vi "MatrixSwitch.vi"(8 "error in (no error)":errorcluster, 10 "Action":T1(ring), 11 "Pickering in":refnum<class "PickeringPrague.lvclass">) -> (0 "error out":errorcluster, 2 "Continue?":bool, 3 "Pickering out":refnum<class "PickeringPrague.lvclass">)   [LabVIEW 2018, in "PickeringPrague.lvclass"]
uses:
  PickeringPrague.lvclass
  InstrumentSetup.vi
  InstrControl.lvclass
panel:
  out "Display Matrix":bool[][](array[boolean])
  # "Pickering Matrix Settings"
  # "X1"
  # "X2"
  # "X3"
  # "X4"
  # "X5"
  # "X6"
  # "X7"
  # "X8"
  # "X9"
  # "X10"
  # "X11"
  # "X12"
  # "Y1"
  # "Y2"
  # "Y3"
  # "Y4"
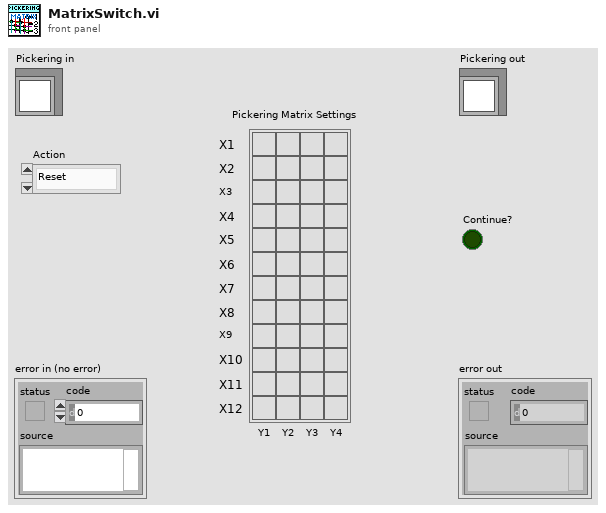
[diagram p1: front panel]
types:
  T1 = enum16{"Reset", "Ground", "Striptest SMU", "Striptest LCR", "IV", "CV", "Interstrip Cap", "Interstrip Res"}
  T2 = cluster{"Matrix address":string, "Mux1 address":string, "Mux2 address":string, "Matrix used?":bool, "Matrix X Channels":cluster{"LCR LO":i32, "LCR HI":i32, "SMU LO":i32, "SMU HI":i32, "GND":i32}, "Matrix Y Channels":cluster{"Flying Probe":i32, "Needle":i32}, "PickeringPrague.lvclass":refnum<class "PickeringPrague.lvclass">}
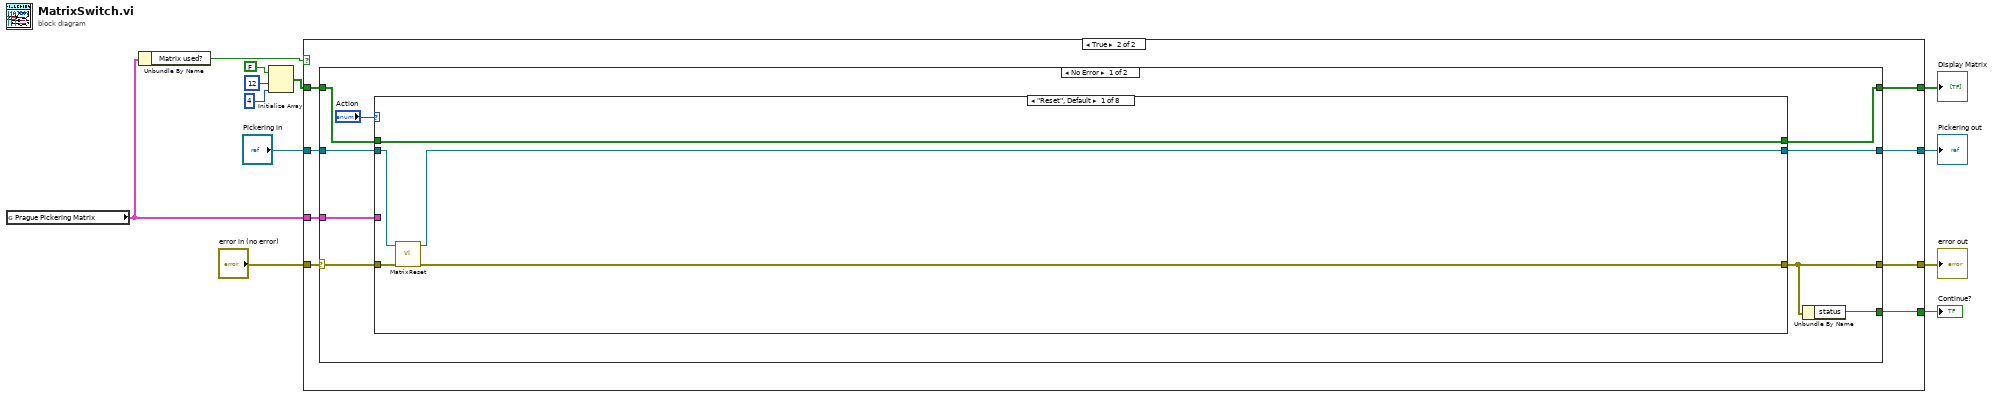
[diagram p0: block diagram]
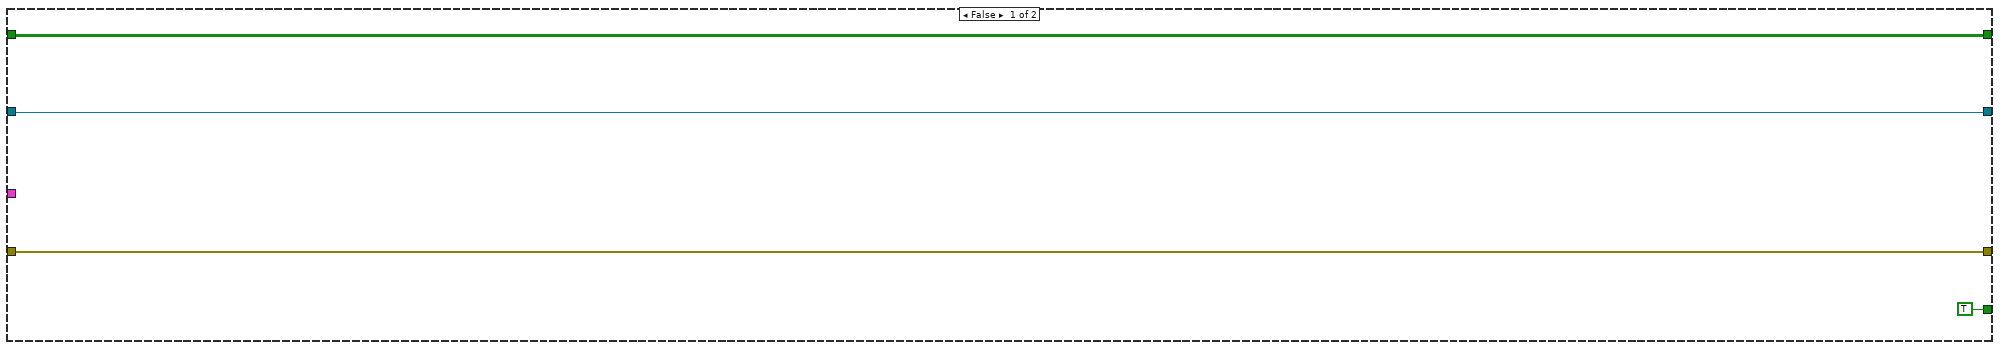
[diagram p2: hidden frame]
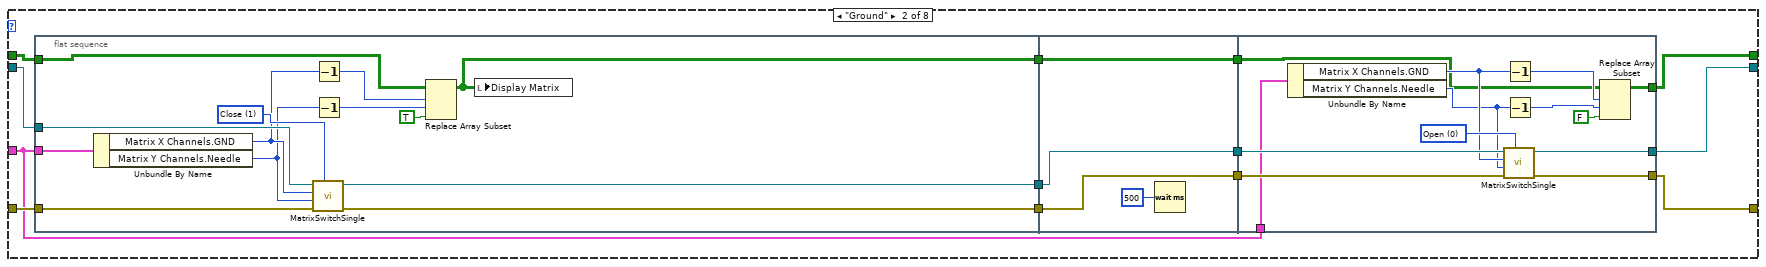
[diagram p3: hidden frame]
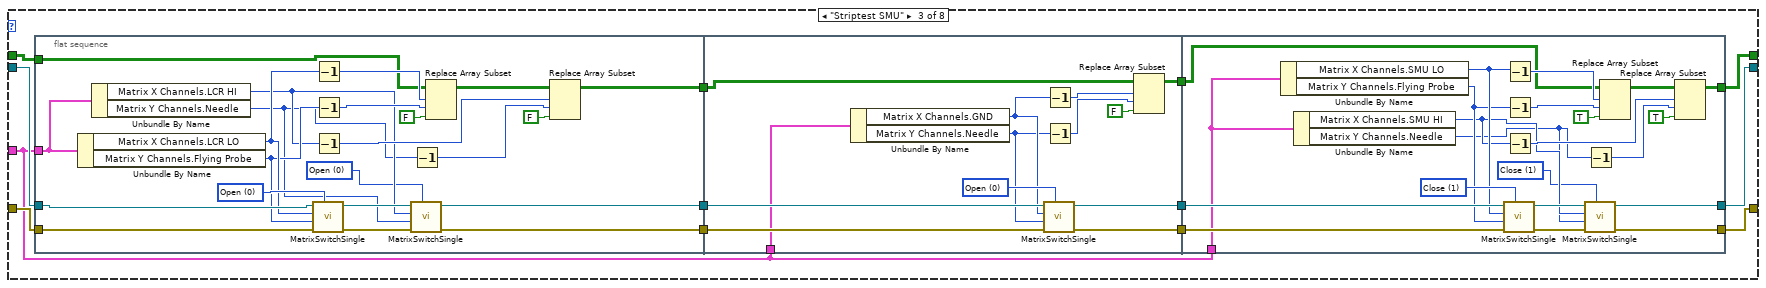
[diagram p4: hidden frame]
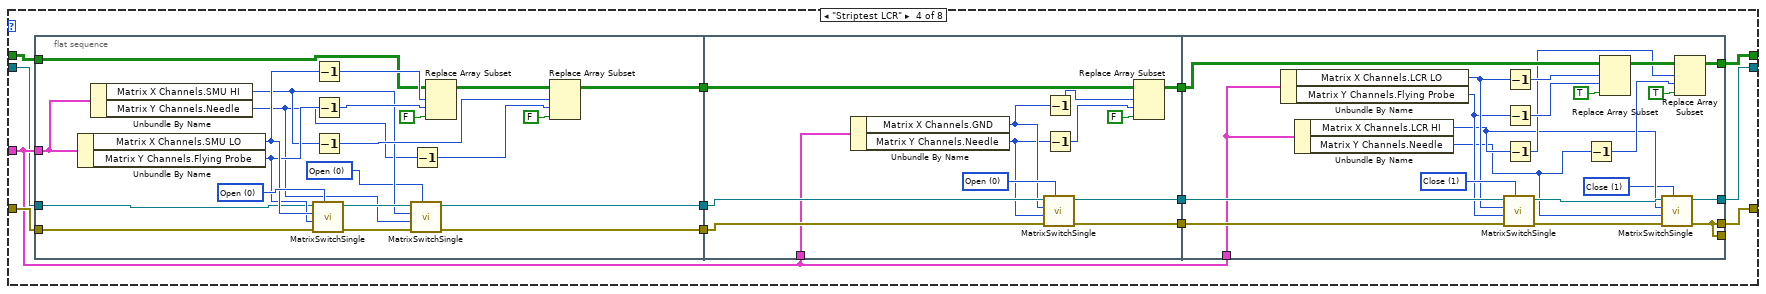
[diagram p5: hidden frame]
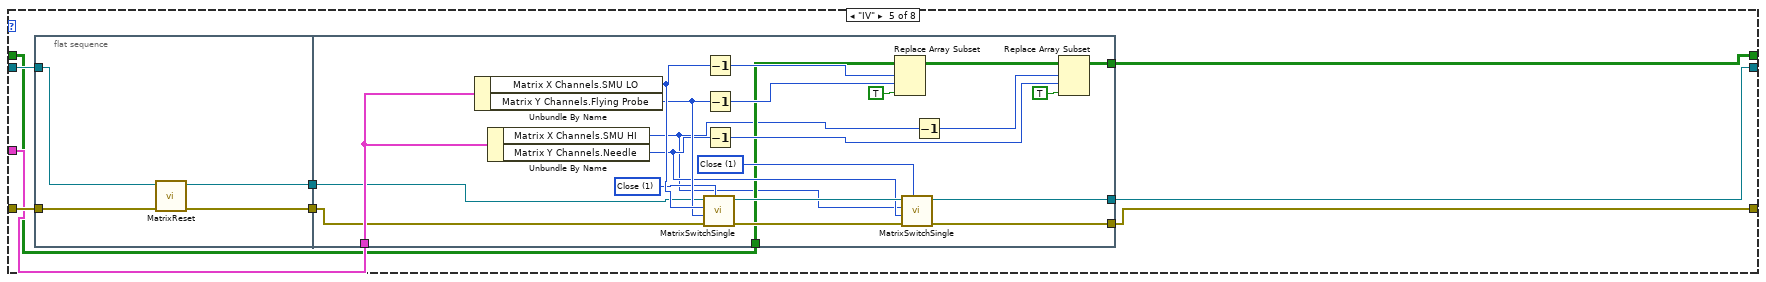
[diagram p6: hidden frame]
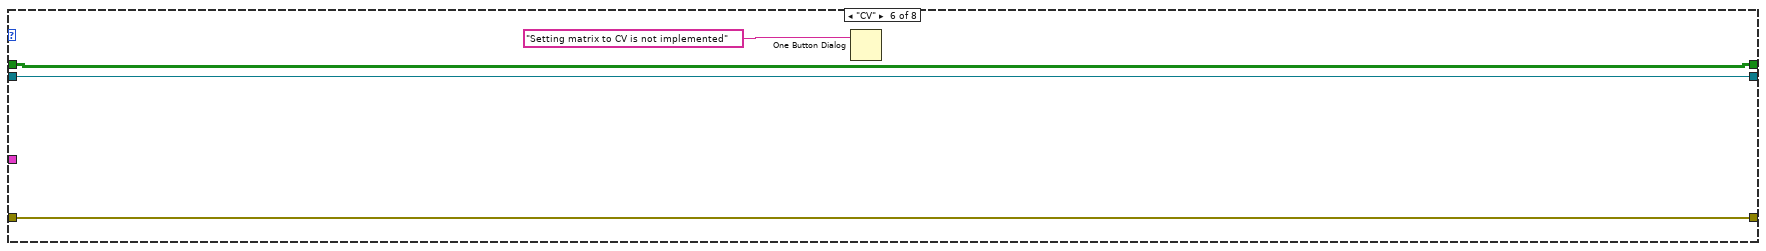
[diagram p7: hidden frame]
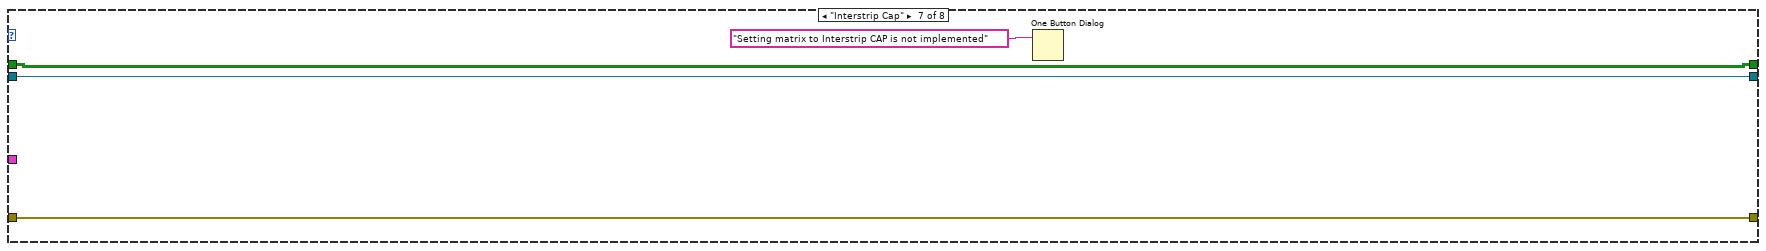
[diagram p8: hidden frame]
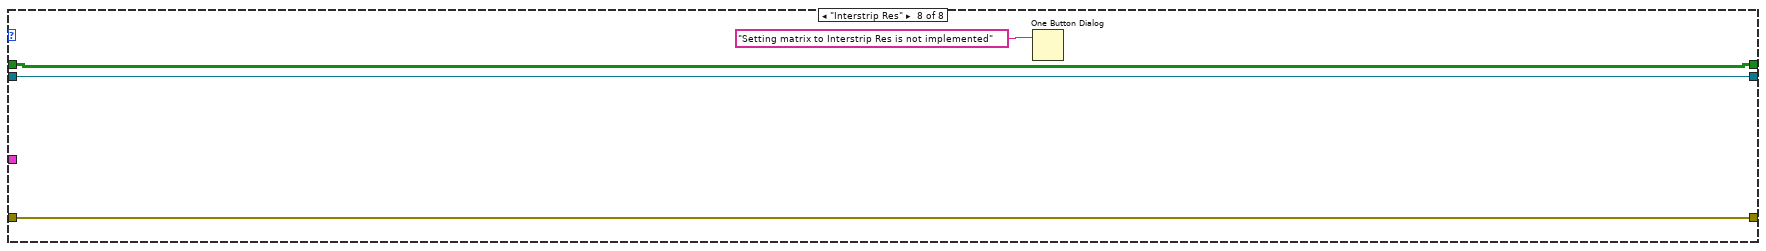
[diagram p9: hidden frame]
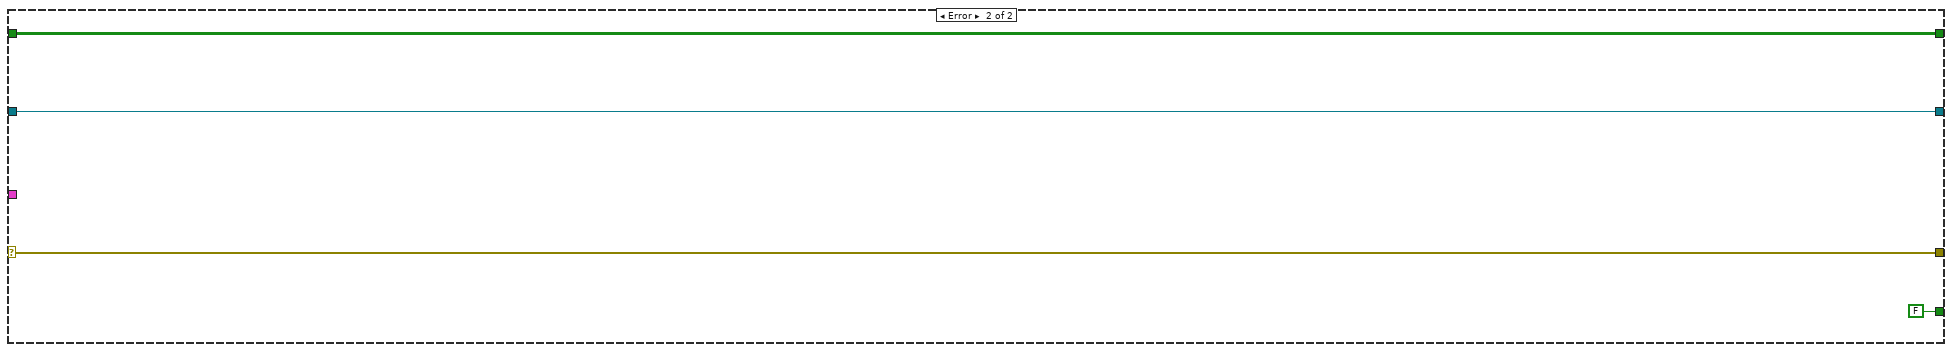
[diagram p10: hidden frame]
diagram:
  n1 = global read "InstrumentSetup.vi" "Prague Pickering Matrix"() -> (w1:T2)
  n2 = Unbundle By Name(w1) -> ("Matrix used?"=w5:bool)
  n3 = Initialize Array(FALSE, 12, 4) -> (w4:bool[][])
  n4 = case shown="True" w5 {
    tunnel: "Pickering in" -> [w16 w24]
    tunnel: "error in (no error)" -> [w15 w23]
    tunnel: w4 -> [w13 w22]
    tunnel: [TRUE ("status") w21] -> w9
    tunnel: [w13 w20] -> w8
    tunnel: [w15 w19] -> w7
    tunnel: [w16 w18] -> w6
    tunnel: w1 -> [_ w17]
    frame False {
    }
    frame True {
      n5 = case shown="No Error" w23 {
        selector: w23 -> [w27 w272]
        tunnel: [w30 w272] -> w19
        tunnel: [w31 w271] -> w18
        tunnel: w24 -> [w28 w271]
        tunnel: [w29 FALSE] -> w21
        tunnel: w22 -> [w33 w269]
        tunnel: [w32 w269] -> w20
        tunnel: w17 -> [w25 _]
        frame No Error {
          n6 = case shown="\"Reset\", Default" "Action" {
            tunnel: w33 -> [w38 w41 w92 w157 w222 w260 w261 w267]
            tunnel: [w38 w43 w84 w153 w224 w260 w261 w267] -> w32
            tunnel: w27 -> [w35 w51 w93 w158 w229 w259 w262 w266]
            tunnel: w28 -> [w37 w48 w94 w152 w230 w258 w263 w265]
            tunnel: [w36 w45 w83 w155 w226 w258 w263 w265] -> w31
            tunnel: [w34 w44 w82 w154 w225 w259 w262 w266] -> w30
            tunnel: w25 -> [_ w42 w85 w156 w223 _ _ _]
            frame "Reset", Default {
              n7 = call-dynamic "MatrixReset.vi"("error in (no error)"=w35, "Pickering in"=w37) -> ("error out"=w34:errorcluster, "Pickering out"=w36:refnum<class "PickeringPrague.lvclass">)  [unwired: 8 in]
            }
            frame "Ground" {
              n8 = flat-sequence {
                tunnel: w51 -> [w63]
                tunnel: [w62] -> w50
                tunnel: w48 -> [w61]
                tunnel: [w60] -> w46
                tunnel: w42 -> [w59]
                tunnel: w41 -> [w54]
                tunnel: [w52] -> w40
                tunnel: w50 -> [w67]
                tunnel: [w67] -> w49
                tunnel: [w66] -> w47
                tunnel: w46 -> [w66]
                tunnel: w40 -> [w65]
                tunnel: [w65] -> w39
                tunnel: w49 -> [w80]
                tunnel: w47 -> [w79]
                tunnel: [w78] -> w45
                tunnel: [w77] -> w44
                tunnel: [w73] -> w43
                tunnel: w42 -> [w72]
                tunnel: w39 -> [w69]
                frame #0 {
                  w64 = u16 1 items=["Open", "Close"] ("Switch action")
                  n9 = Unbundle By Name(w59) -> ("Matrix X Channels.GND"=w58:i32, "Matrix Y Channels.Needle"=w55:i32)
                  n10 = call-dynamic "MatrixSwitchSingle.vi"("Switch action"=w64, "error in (no error)"=w63, "Matrix Y"=w55, "Matrix X"=w58, "Pickering in"=w61) -> ("error out"=w62:errorcluster, "Pickering out"=w60:refnum<class "PickeringPrague.lvclass">)  [unwired: 4 in, 1 out]
                  n11 = Decrement(x=w58) -> (x-1=w57:i32)
                  n12 = Decrement(x=w55) -> (x-1=w56:i32)
                  n13 = Replace Array Subset(array=w54, new element=TRUE ("new element/subarray"), index (row)=w57, index (col)=w56) -> (w52:bool[][])
                  n14 = local write "Display Matrix"(w52) -> ()
                }
                frame #1 {
                  n15 = Wait (ms)(milliseconds to wait=u32 500) -> ()  [unwired: 1 out]
                }
                frame #2 {
                  w81 = u16 0 items=["Open", "Close"] ("Switch action")
                  n16 = Unbundle By Name(w72) -> ("Matrix X Channels.GND"=w71:i32, "Matrix Y Channels.Needle"=w70:i32)
                  n17 = call-dynamic "MatrixSwitchSingle.vi"("Switch action"=w81, "error in (no error)"=w80, "Matrix Y"=w70, "Matrix X"=w71, "Pickering in"=w79) -> ("error out"=w77:errorcluster, "Pickering out"=w78:refnum<class "PickeringPrague.lvclass">)  [unwired: 4 in, 1 out]
                  n18 = Decrement(x=w71) -> (x-1=w75:i32)
                  n19 = Decrement(x=w70) -> (x-1=w76:i32)
                  n20 = Replace Array Subset(array=w69, new element=FALSE ("new element/subarray"), index (row)=w75, index (col)=w76) -> (w73:bool[][])
                }
              }
            }
            frame "Striptest SMU" {
              n21 = flat-sequence {
                tunnel: w94 -> [w116]
                tunnel: w93 -> [w115]
                tunnel: w85 -> [w112]
                tunnel: [w111] -> w91
                tunnel: [w110] -> w90
                tunnel: w92 -> [w104]
                tunnel: [w95] -> w87
                tunnel: w91 -> [w126]
                tunnel: w90 -> [w129]
                tunnel: [w128] -> w89
                tunnel: [w127] -> w88
                tunnel: w87 -> [w119]
                tunnel: w85 -> [w118]
                tunnel: [w117] -> w86
                tunnel: w89 -> [w151]
                tunnel: w88 -> [w149]
                tunnel: w85 -> [w130]
                tunnel: w86 -> [w144]
                tunnel: [w133] -> w84
                tunnel: [w132] -> w83
                tunnel: [w131] -> w82
                frame #0 {
                  w96 = u16 0 items=["Open", "Close"] ("Switch action")
                  w109 = u16 0 items=["Open", "Close"] ("Switch action")
                  n22 = Unbundle By Name(w112) -> ("Matrix X Channels.LCR LO"=w106:i32, "Matrix Y Channels.Flying Probe"=w105:i32)
                  n23 = Unbundle By Name(w112) -> ("Matrix X Channels.LCR HI"=w99:i32, "Matrix Y Channels.Needle"=w98:i32)
                  n24 = call-dynamic "MatrixSwitchSingle.vi"("Switch action"=w109, "error in (no error)"=w115, "Matrix Y"=w105, "Matrix X"=w106, "Pickering in"=w116) -> ("error out"=w114:errorcluster, "Pickering out"=w113:refnum<class "PickeringPrague.lvclass">)  [unwired: 4 in, 1 out]
                  n25 = Decrement(x=w106) -> (x-1=w108:i32)
                  n26 = Decrement(x=w105) -> (x-1=w107:i32)
                  n27 = Decrement(x=w99) -> (x-1=w100:i32)
                  n28 = call-dynamic "MatrixSwitchSingle.vi"("Switch action"=w96, "error in (no error)"=w114, "Matrix Y"=w98, "Matrix X"=w99, "Pickering in"=w113) -> ("error out"=w111:errorcluster, "Pickering out"=w110:refnum<class "PickeringPrague.lvclass">)  [unwired: 4 in, 1 out]
                  n29 = Decrement(x=w98) -> (x-1=w101:i32)
                  n30 = Replace Array Subset(array=w104, new element=FALSE, index (row)=w108, index (col)=w107) -> (w102:bool[][])
                  n31 = Replace Array Subset(array=w102, new element=FALSE, index (row)=w100, index (col)=w101) -> (w95:bool[][])
                }
                frame #1 {
                  w125 = u16 0 items=["Open", "Close"] ("Switch action")
                  n32 = Unbundle By Name(w118) -> ("Matrix X Channels.GND"=w121:i32, "Matrix Y Channels.Needle"=w120:i32)
                  n33 = call-dynamic "MatrixSwitchSingle.vi"("Switch action"=w125, "error in (no error)"=w126, "Matrix Y"=w120, "Matrix X"=w121, "Pickering in"=w129) -> ("error out"=w127:errorcluster, "Pickering out"=w128:refnum<class "PickeringPrague.lvclass">)  [unwired: 4 in, 1 out]
                  n34 = Decrement(x=w121) -> (x-1=w123:i32)
                  n35 = Decrement(x=w120) -> (x-1=w122:i32)
                  n36 = Replace Array Subset(array=w119, new element=FALSE, index (row)=w123, index (col)=w122) -> (w117:bool[][])
                }
                frame #2 {
                  w134 = u16 1 items=["Open", "Close"] ("Switch action")
                  w147 = u16 1 items=["Open", "Close"] ("Switch action")
                  n37 = Unbundle By Name(w130) -> ("Matrix X Channels.SMU LO"=w142:i32, "Matrix Y Channels.Flying Probe"=w141:i32)
                  n38 = Unbundle By Name(w130) -> ("Matrix X Channels.SMU HI"=w137:i32, "Matrix Y Channels.Needle"=w136:i32)
                  n39 = call-dynamic "MatrixSwitchSingle.vi"("Switch action"=w147, "error in (no error)"=w149, "Matrix Y"=w141, "Matrix X"=w142, "Pickering in"=w151) -> ("error out"=w148:errorcluster, "Pickering out"=w150:refnum<class "PickeringPrague.lvclass">)  [unwired: 4 in, 1 out]
                  n40 = Decrement(x=w142) -> (x-1=w146:i32)
                  n41 = Decrement(x=w141) -> (x-1=w145:i32)
                  n42 = Decrement(x=w137) -> (x-1=w139:i32)
                  n43 = call-dynamic "MatrixSwitchSingle.vi"("Switch action"=w134, "error in (no error)"=w148, "Matrix Y"=w136, "Matrix X"=w137, "Pickering in"=w150) -> ("error out"=w131:errorcluster, "Pickering out"=w132:refnum<class "PickeringPrague.lvclass">)  [unwired: 4 in, 1 out]
                  n44 = Decrement(x=w136) -> (x-1=w138:i32)
                  n45 = Replace Array Subset(array=w144, new element=TRUE ("new element/subarray"), index (row)=w146, index (col)=w145) -> (w140:bool[][])
                  n46 = Replace Array Subset(array=w140, new element=TRUE ("new element/subarray"), index (row)=w139, index (col)=w138) -> (w133:bool[][])
                }
              }
            }
            frame "Striptest LCR" {
              n47 = flat-sequence {
                tunnel: w158 -> [w186]
                tunnel: w156 -> [w183]
                tunnel: [w182] -> w164
                tunnel: [w181] -> w163
                tunnel: w157 -> [w175]
                tunnel: [w166] -> w162
                tunnel: w152 -> [w165]
                tunnel: w164 -> [w196]
                tunnel: w163 -> [w199]
                tunnel: [w198] -> w161
                tunnel: [w197] -> w160
                tunnel: w162 -> [w189]
                tunnel: w156 -> [w188]
                tunnel: [w187] -> w159
                tunnel: w161 -> [w221]
                tunnel: w160 -> [w219]
                tunnel: w156 -> [w201]
                tunnel: w159 -> [w214]
                tunnel: [w203] -> w153
                tunnel: [w202] -> w155
                tunnel: [w200] -> _
                tunnel: [w200] -> w154
                frame #0 {
                  w167 = u16 0 items=["Open", "Close"] ("Switch action")
                  w180 = u16 0 items=["Open", "Close"] ("Switch action")
                  n48 = Unbundle By Name(w183) -> ("Matrix X Channels.SMU LO"=w177:i32, "Matrix Y Channels.Flying Probe"=w176:i32)
                  n49 = Unbundle By Name(w183) -> ("Matrix X Channels.SMU HI"=w170:i32, "Matrix Y Channels.Needle"=w169:i32)
                  n50 = call-dynamic "MatrixSwitchSingle.vi"("Switch action"=w180, "error in (no error)"=w186, "Matrix Y"=w176, "Matrix X"=w177, "Pickering in"=w165) -> ("error out"=w185:errorcluster, "Pickering out"=w184:refnum<class "PickeringPrague.lvclass">)  [unwired: 4 in, 1 out]
                  n51 = Decrement(x=w177) -> (x-1=w179:i32)
                  n52 = Decrement(x=w176) -> (x-1=w178:i32)
                  n53 = Decrement(x=w170) -> (x-1=w171:i32)
                  n54 = call-dynamic "MatrixSwitchSingle.vi"("Switch action"=w167, "error in (no error)"=w185, "Matrix Y"=w169, "Matrix X"=w170, "Pickering in"=w184) -> ("error out"=w182:errorcluster, "Pickering out"=w181:refnum<class "PickeringPrague.lvclass">)  [unwired: 4 in, 1 out]
                  n55 = Decrement(x=w169) -> (x-1=w172:i32)
                  n56 = Replace Array Subset(array=w175, new element=FALSE, index (row)=w179, index (col)=w178) -> (w173:bool[][])
                  n57 = Replace Array Subset(array=w173, new element=FALSE, index (row)=w171, index (col)=w172) -> (w166:bool[][])
                }
                frame #1 {
                  w195 = u16 0 items=["Open", "Close"] ("Switch action")
                  n58 = Unbundle By Name(w188) -> ("Matrix X Channels.GND"=w191:i32, "Matrix Y Channels.Needle"=w190:i32)
                  n59 = call-dynamic "MatrixSwitchSingle.vi"("Switch action"=w195, "error in (no error)"=w196, "Matrix Y"=w190, "Matrix X"=w191, "Pickering in"=w199) -> ("error out"=w197:errorcluster, "Pickering out"=w198:refnum<class "PickeringPrague.lvclass">)  [unwired: 4 in, 1 out]
                  n60 = Decrement(x=w191) -> (x-1=w193:i32)
                  n61 = Decrement(x=w190) -> (x-1=w192:i32)
                  n62 = Replace Array Subset(array=w189, new element=FALSE, index (row)=w193, index (col)=w192) -> (w187:bool[][])
                }
                frame #2 {
                  w204 = u16 1 items=["Open", "Close"] ("Switch action")
                  w217 = u16 1 items=["Open", "Close"] ("Switch action")
                  n63 = Unbundle By Name(w201) -> ("Matrix X Channels.LCR LO"=w212:i32, "Matrix Y Channels.Flying Probe"=w211:i32)
                  n64 = Unbundle By Name(w201) -> ("Matrix X Channels.LCR HI"=w207:i32, "Matrix Y Channels.Needle"=w206:i32)
                  n65 = call-dynamic "MatrixSwitchSingle.vi"("Switch action"=w217, "error in (no error)"=w219, "Matrix Y"=w211, "Matrix X"=w212, "Pickering in"=w221) -> ("error out"=w218:errorcluster, "Pickering out"=w220:refnum<class "PickeringPrague.lvclass">)  [unwired: 4 in, 1 out]
                  n66 = Decrement(x=w212) -> (x-1=w216:i32)
                  n67 = Decrement(x=w211) -> (x-1=w215:i32)
                  n68 = Decrement(x=w207) -> (x-1=w209:i32)
                  n69 = Decrement(x=w206) -> (x-1=w208:i32)
                  n70 = Replace Array Subset(array=w214, new element=TRUE ("new element/subarray"), index (row)=w216, index (col)=w215) -> (w210:bool[][])
                  n71 = call-dynamic "MatrixSwitchSingle.vi"("Switch action"=w204, "error in (no error)"=w218, "Matrix Y"=w206, "Matrix X"=w207, "Pickering in"=w220) -> ("error out"=w200:errorcluster, "Pickering out"=w202:refnum<class "PickeringPrague.lvclass">)  [unwired: 4 in, 1 out]
                  n72 = Replace Array Subset(array=w210, new element=TRUE ("new element/subarray"), index (row)=w209, index (col)=w208) -> (w203:bool[][])
                }
              }
            }
            frame "IV" {
              n73 = flat-sequence {
                tunnel: w230 -> [w234]
                tunnel: w229 -> [w233]
                tunnel: [w232] -> w228
                tunnel: [w231] -> w227
                tunnel: w228 -> [w241]
                tunnel: w227 -> [w240]
                tunnel: [w238] -> w226
                tunnel: [w239] -> w225
                tunnel: [w236] -> w224
                tunnel: w223 -> [w242]
                tunnel: w222 -> [w237]
                frame #0 {
                  n74 = call-dynamic "MatrixReset.vi"("error in (no error)"=w233, "Pickering in"=w234) -> ("error out"=w231:errorcluster, "Pickering out"=w232:refnum<class "PickeringPrague.lvclass">)  [unwired: 8 in]
                }
                frame #1 {
                  w245 = u16 1 items=["Open", "Close"] ("Switch action")
                  w243 = u16 1 items=["Open", "Close"] ("Switch action")
                  n75 = Unbundle By Name(w242) -> ("Matrix X Channels.SMU LO"=w252:i32, "Matrix Y Channels.Flying Probe"=w251:i32)
                  n76 = Unbundle By Name(w242) -> ("Matrix X Channels.SMU HI"=w235:i32, "Matrix Y Channels.Needle"=w247:i32)
                  n77 = call-dynamic "MatrixSwitchSingle.vi"("Switch action"=w243, "error in (no error)"=w240, "Matrix Y"=w251, "Matrix X"=w252, "Pickering in"=w241) -> ("error out"=w255:errorcluster, "Pickering out"=w256:refnum<class "PickeringPrague.lvclass">)  [unwired: 4 in, 1 out]
                  n78 = Decrement(x=w252) -> (x-1=w254:i32)
                  n79 = Decrement(x=w251) -> (x-1=w253:i32)
                  n80 = Decrement(x=w247) -> (x-1=w248:i32)
                  n81 = Replace Array Subset(array=w237, new element=TRUE ("new element/subarray"), index (row)=w254, index (col)=w253) -> (w250:bool[][])
                  n82 = call-dynamic "MatrixSwitchSingle.vi"("Switch action"=w245, "error in (no error)"=w255, "Matrix Y"=w247, "Matrix X"=w235, "Pickering in"=w256) -> ("error out"=w239:errorcluster, "Pickering out"=w238:refnum<class "PickeringPrague.lvclass">)  [unwired: 4 in, 1 out]
                  n83 = Decrement(x=w235) -> (x-1=w249:i32)
                  n84 = Replace Array Subset(array=w250, new element=TRUE ("new element/subarray"), index (row)=w249, index (col)=w248) -> (w236:bool[][])
                }
              }
            }
            frame "CV" {
              n85 = One Button Dialog(message="Setting matrix to CV is not implemented") -> ()  [unwired: 1 in, 1 out]
            }
            frame "Interstrip Cap" {
              n86 = One Button Dialog(message="Setting matrix to Interstrip CAP is not implemented") -> ()  [unwired: 1 in, 1 out]
            }
            frame "Interstrip Res" {
              n87 = One Button Dialog(message="Setting matrix to Interstrip Res is not implemented") -> ()  [unwired: 1 in, 1 out]
            }
          }
          n88 = Unbundle By Name(w30) -> ("status"=w29:bool)
        }
        frame Error {
        }
      }
    }
  }
  "error out" <- w7
  "Pickering out" <- w6
  "Display Matrix" <- w8
  "Continue?" <- w9
